vi "PH_Beckhoff-16BB_Testtool.ProcPeriodic.vi"(0 "i ref in":refnum<vi>, 3 "ms timeout (100)":i32=100, 5 "error in (no error)":errorcluster) -> (14 "i ref out":refnum<vi>, 17 "timed out":bool, 19 "error out":errorcluster)   [LabVIEW 2014, in "PH_Beckhoff-16BB_Testtool.lvlib"]
doc: "This method serves to periodically do things like reading values from the HW. Methods that should be executed periodically should be called from THIS methode. Add code here."
uses:
  PH_Beckhoff-16BB_Testtool.lvlib
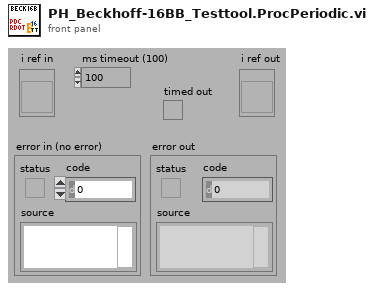
[diagram p1: front panel]
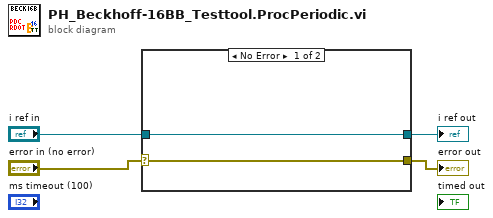
[diagram p0: block diagram]
diagram:
  n1 = case shown="No Error" "error in (no error)" {
    selector: "error in (no error)" -> [w5 w7]
    tunnel: [w5 w7] -> w4
    tunnel: [w6 w8] -> w3
    tunnel: "i ref in" -> [w6 w8]
    frame No Error {
    }
    frame Error {
    }
  }
  "error out" <- w4
  "i ref out" <- w3
